vi "E727_StageNavigator.vi"() -> ()   [LabVIEW 2022 SP3]
panel:
  in  "stop":bool
  out "Current position":dbl[](array[numeric]) format="%.6f"
  out "StageRunning":bool
  in  "Repeats":dbl=1.0 min=1.0
  in  "Left x0.5":bool
  in  "Right x0.5":bool
  in  "Up x0.5":bool
  in  "Down x0.5":bool
  in  "Z Resolution (um)":dbl=30.0 min=1.0
  in  "Down Z x4":bool
  in  "Down Z x2":bool
  in  "Up Z x4":bool
  in  "Up Z x2":bool
  in  "Up Z":bool
  in  "Down Z":bool
  in  "Right x4":bool
  in  "Right x2":bool
  in  "Left x4":bool
  in  "Left x2":bool
  in  "Down x4":bool
  in  "Down x2":bool
  in  "Up x4":bool
  in  "Up x2":bool
  in  "StageChannels":string[](array[string])
  in  "On/Off":bool
  in  "X / Y Resolution (um)":dbl=10.0 min=1.0
  in  "Right":bool
  in  "Left":bool
  in  "Up":bool
  in  "Down":bool
  # "STAGE"
  # "Z Focus"
  # "X / Y Navigation"
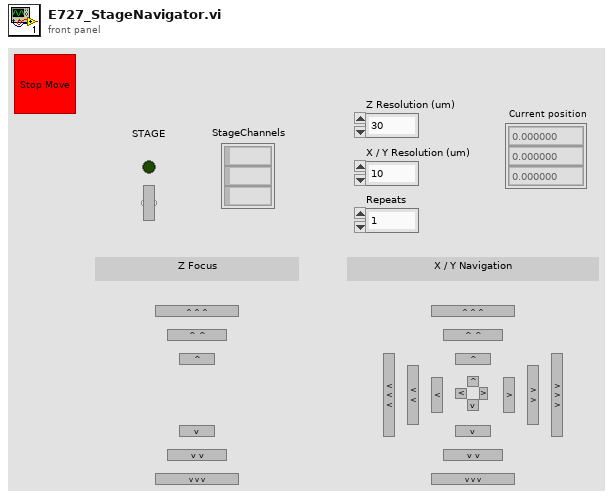
[diagram p1: front panel]
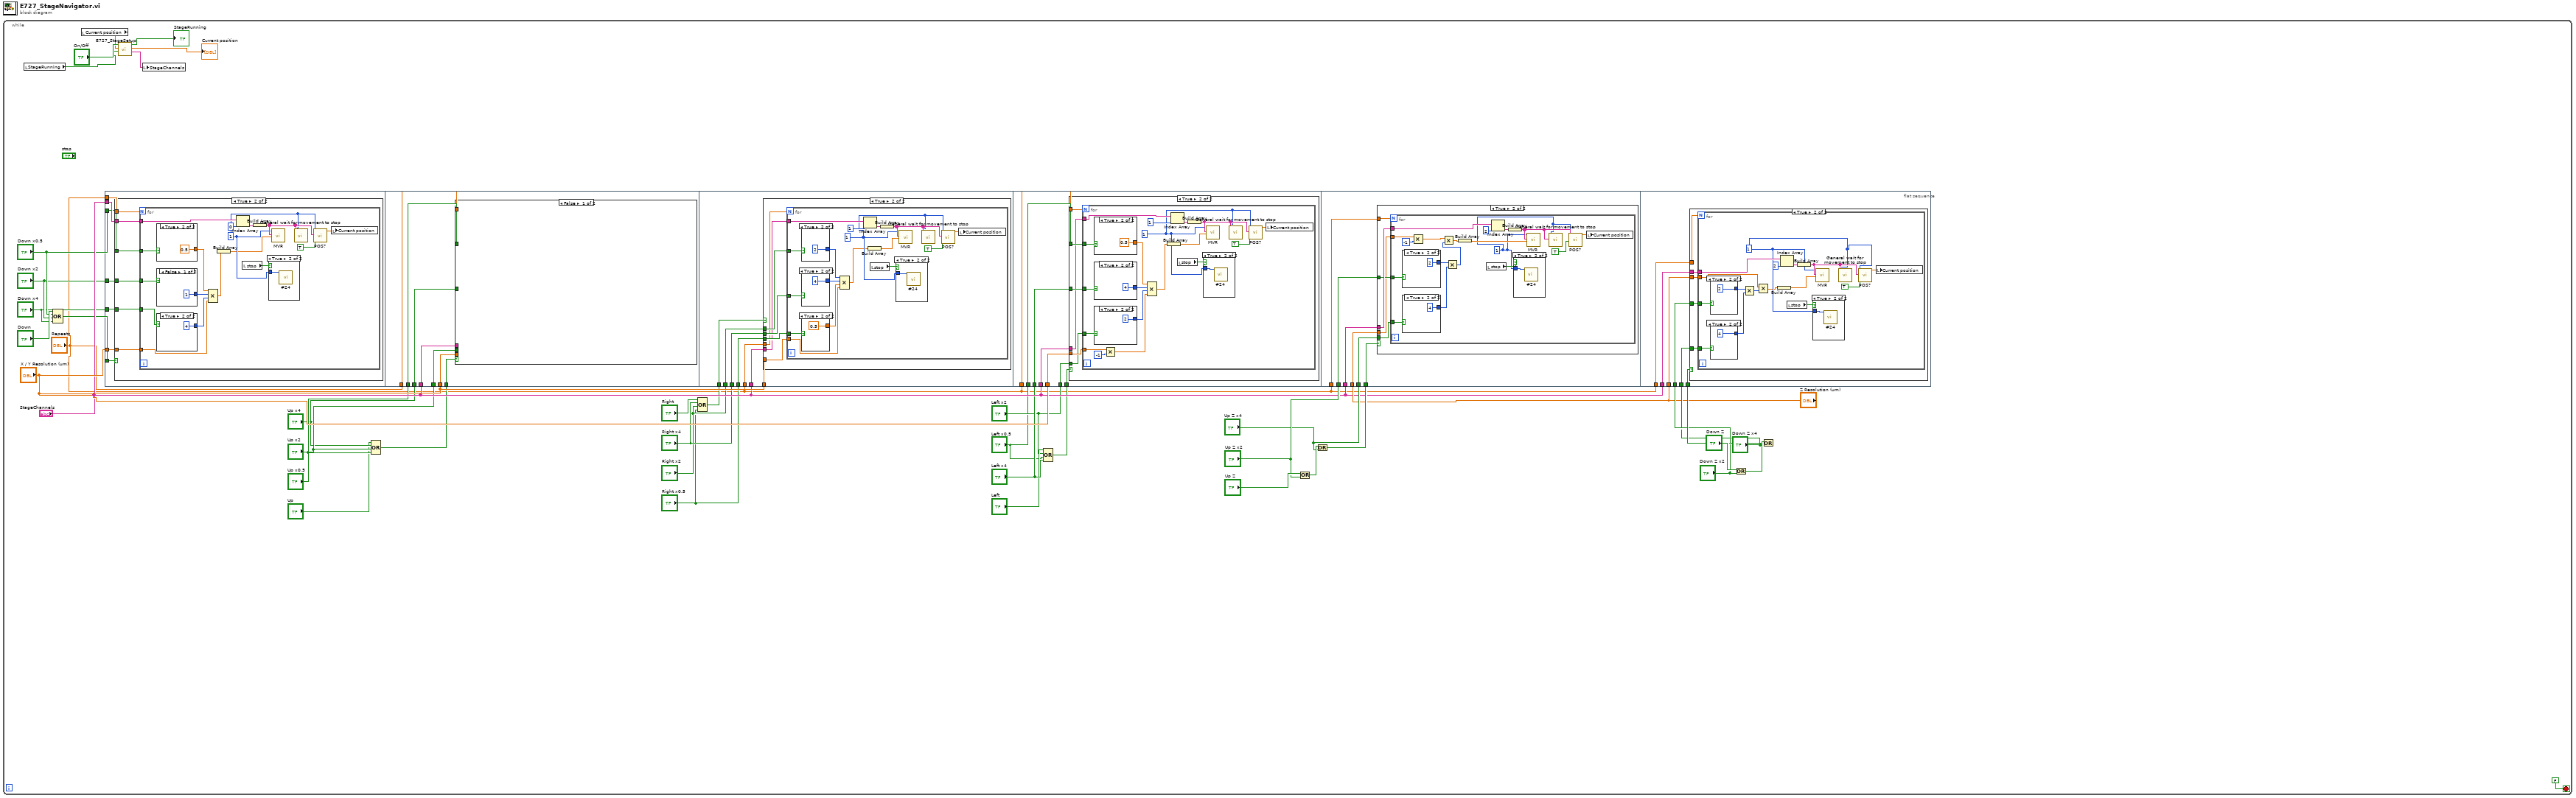
[diagram p0: block diagram]
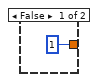
[diagram p4: hidden frame]
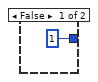
[diagram p5: hidden frame]
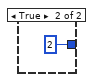
[diagram p6: hidden frame]
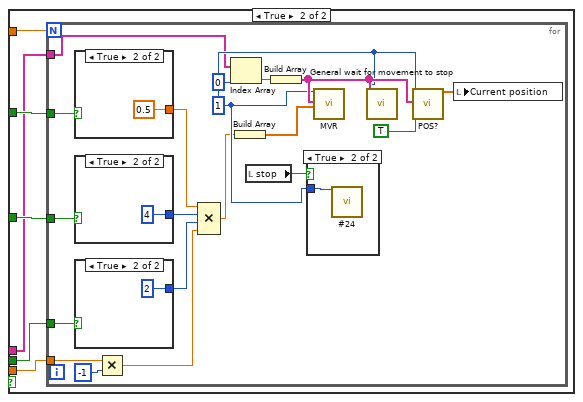
[diagram p7: hidden frame]
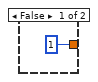
[diagram p9: hidden frame]
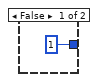
[diagram p10: hidden frame]
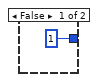
[diagram p11: hidden frame]
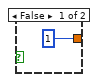
[diagram p14: hidden frame]
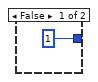
[diagram p15: hidden frame]
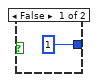
[diagram p16: hidden frame]
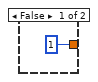
[diagram p19: hidden frame]
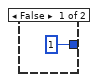
[diagram p20: hidden frame]
diagram:
  n1 = while {
    stop <- FALSE stop-if-true
    n2 = local read "StageRunning"() -> (w5:bool)
    n3 = Compound Arithmetic op=OR("Down", "Down x0.5", "Down x2", "Down x4") -> (w13:bool)
    n4 = local read "Current position"() -> (w1:dbl[])
    n5 = flat-sequence {
      tunnel: "X / Y Resolution (um)" -> [w47]
      tunnel: "StageChannels" -> [w48]
      tunnel: w13 -> [w46]
      tunnel: "Down x2" -> [w45]
      tunnel: "Down x4" -> [w44]
      tunnel: "Down x0.5" -> [w43]
      tunnel: "Repeats" -> [w42]
      tunnel: "X / Y Resolution (um)" -> [w85]
      tunnel: "StageChannels" -> [w84]
      tunnel: "Up x2" -> [w83]
      tunnel: w18 -> [w82]
      tunnel: "Up x4" -> [w81]
      tunnel: "Up x0.5" -> [w80]
      tunnel: "Repeats" -> [w79]
      tunnel: "StageChannels" -> [w124]
      tunnel: "Right x2" -> [w123]
      tunnel: "Right x4" -> [w122]
      tunnel: "X / Y Resolution (um)" -> [w121]
      tunnel: w28 -> [w120]
      tunnel: "Right x0.5" -> [w119]
      tunnel: "Repeats" -> [w118]
      tunnel: "StageChannels" -> [w161]
      tunnel: "X / Y Resolution (um)" -> [w160]
      tunnel: w23 -> [w159]
      tunnel: "Left x4" -> [w158]
      tunnel: "Left x2" -> [w157]
      tunnel: "Left x0.5" -> [w156]
      tunnel: "Repeats" -> [w155]
      tunnel: "StageChannels" -> [w199]
      tunnel: "Z Resolution (um)" -> [w198]
      tunnel: w39 -> [w197]
      tunnel: "Up Z x2" -> [w196]
      tunnel: "Up Z x4" -> [w195]
      tunnel: "Repeats" -> [w194]
      tunnel: "StageChannels" -> [w233]
      tunnel: "Z Resolution (um)" -> [w232]
      tunnel: w33 -> [w231]
      tunnel: "Down Z x2" -> [w230]
      tunnel: "Down Z x4" -> [w229]
      tunnel: "Repeats" -> [w228]
      frame #0 {
        n6 = case shown="True" w46 {
          tunnel: w47 -> [_ w51]
          tunnel: w48 -> [_ w54]
          tunnel: w45 -> [_ w53]
          tunnel: w44 -> [_ w52]
          tunnel: w43 -> [_ w50]
          tunnel: w42 -> [_ w49]
          frame False {
          }
          frame True {
            n7 = for {
              N: w49 -> [_]
              tunnel: w54 -> [w58]
              tunnel: w53 -> [w71]
              tunnel: w52 -> [w70]
              tunnel: w51 -> [w69]
              tunnel: w50 -> [w65]
              w57 = 1 ("System no.")
              n8 = case shown="True" w65 {
                tunnel: [1 0.5] -> w68
                frame False {
                }
                frame True {
                }
              }
              n9 = case shown="False" w71 {
                tunnel: [1 2] -> w66
                frame False {
                }
                frame True {
                }
              }
              n10 = case shown="True" w70 {
                tunnel: [1 4] -> w67
                frame False {
                }
                frame True {
                }
              }
              n11 = Compound Arithmetic op=MULTIPLY(w68, w66, w67, w69) -> (w56:dbl)
              n12 = Build Array(w56) -> (w55:dbl[])
              n13 = Index Array(array=w58, index=0) -> (element=w61:string)
              n14 = local read "stop"() -> (w62:bool)
              n15 = Build Array(w61) -> (w63:string[])
              n16 = case shown="True" w62 {
                tunnel: w57 -> [_ w72]
                frame False {
                }
                frame True {
                  n17 = call "#24.vi"("System no."=w72) -> ()  [unwired: 1 in, 18 out]
                }
              }
              n18 = call "MVR.vi"("System no."=w57, "Axes to move"=w63, "Position values"=w55) -> ()  [unwired: 2 in, 15 out]
              n19 = call "General wait for movement to stop.vi"("System no."=w57, "Axes to wait for"=w63) -> ()  [unwired: 6 in, 12 out]
              n20 = call "POS?.vi"("System no."=w57, "Axes to query"=w63, "All axes?"=TRUE) -> ("Position"=w64:dbl[])  [unwired: 2 in, 14 out]
              n21 = local write "Current position"(w64) -> ()
            }
          }
        }
      }
      frame #1 {
        n22 = case shown="False" w82 {
          tunnel: w85 -> [_ w91]
          tunnel: w84 -> [_ w87]
          tunnel: w83 -> [_ w90]
          tunnel: w81 -> [_ w89]
          tunnel: w80 -> [_ w88]
          tunnel: w79 -> [_ w86]
          frame False {
          }
          frame True {
            n23 = for {
              N: w86 -> [_]
              tunnel: w91 -> [w102]
              tunnel: w90 -> [w109]
              tunnel: w89 -> [w108]
              tunnel: w88 -> [w103]
              tunnel: w87 -> [w94]
              w95 = 1 ("System no.")
              n24 = case shown="True" w103 {
                tunnel: [1 0.5] -> w106
                frame False {
                }
                frame True {
                }
              }
              n25 = case shown="True" w108 {
                tunnel: [1 4] -> w105
                frame False {
                }
                frame True {
                }
              }
              n26 = case shown="True" w109 {
                tunnel: [1 2] -> w104
                frame False {
                }
                frame True {
                }
              }
              n27 = Multiply(x=w102, y=-1) -> (x*y=w107:dbl)
              n28 = Compound Arithmetic op=MULTIPLY(w106, w105, w104, w107) -> (w92:dbl)
              n29 = Index Array(array=w94, index=0) -> (element=w98:string)
              n30 = Build Array(w92) -> (w93:dbl[])
              n31 = local read "stop"() -> (w99:bool)
              n32 = Build Array(w98) -> (w100:string[])
              n33 = case shown="True" w99 {
                tunnel: w95 -> [_ w111]
                frame False {
                }
                frame True {
                  n34 = call "#24.vi"("System no."=w111) -> ()  [unwired: 1 in, 18 out]
                }
              }
              n35 = call "MVR.vi"("System no."=w95, "Axes to move"=w100, "Position values"=w93) -> ()  [unwired: 2 in, 15 out]
              n36 = call "General wait for movement to stop.vi"("System no."=w95, "Axes to wait for"=w100) -> ()  [unwired: 6 in, 12 out]
              n37 = call "POS?.vi"("System no."=w95, "Axes to query"=w100, "All axes?"=TRUE) -> ("Position"=w101:dbl[])  [unwired: 2 in, 14 out]
              n38 = local write "Current position"(w101) -> ()
            }
          }
        }
      }
      frame #2 {
        n39 = case shown="True" w120 {
          tunnel: w121 -> [_ w127]
          tunnel: w124 -> [_ w126]
          tunnel: w123 -> [_ w130]
          tunnel: w122 -> [_ w129]
          tunnel: w119 -> [_ w128]
          tunnel: w118 -> [_ w125]
          frame False {
          }
          frame True {
            n40 = for {
              N: w125 -> [_]
              tunnel: w130 -> [w147]
              tunnel: w129 -> [w146]
              tunnel: w128 -> [w144]
              tunnel: w127 -> [w141]
              tunnel: w126 -> [w135]
              w133 = 1 ("System no.")
              n41 = case shown="True" w147 {
                tunnel: [1 2] -> w143
                frame False {
                }
                frame True {
                }
              }
              n42 = case shown="True" w146 {
                tunnel: [1 4] -> w142
                frame False {
                }
                frame True {
                }
              }
              n43 = case shown="True" w144 {
                tunnel: [1 0.5] -> w145
                frame False {
                }
                frame True {
                }
              }
              n44 = Compound Arithmetic op=MULTIPLY(w143, w142, w145, w141) -> (w131:dbl)
              n45 = Index Array(array=w135, index=1) -> (element=w137:string)
              n46 = Build Array(w131) -> (w132:dbl[])
              n47 = local read "stop"() -> (w138:bool)
              n48 = Build Array(w137) -> (w139:string[])
              n49 = case shown="True" w138 {
                tunnel: w133 -> [_ w148]
                frame False {
                }
                frame True {
                  n50 = call "#24.vi"("System no."=w148) -> ()  [unwired: 1 in, 18 out]
                }
              }
              n51 = call "MVR.vi"("System no."=w133, "Axes to move"=w139, "Position values"=w132) -> ()  [unwired: 2 in, 15 out]
              n52 = call "General wait for movement to stop.vi"("System no."=w133, "Axes to wait for"=w139) -> ()  [unwired: 6 in, 12 out]
              n53 = call "POS?.vi"("System no."=w133, "Axes to query"=w139, "All axes?"=TRUE) -> ("Position"=w140:dbl[])  [unwired: 2 in, 14 out]
              n54 = local write "Current position"(w140) -> ()
            }
          }
        }
      }
      frame #3 {
        n55 = case shown="True" w159 {
          tunnel: w160 -> [_ w167]
          tunnel: w161 -> [_ w163]
          tunnel: w157 -> [_ w166]
          tunnel: w158 -> [_ w165]
          tunnel: w156 -> [_ w164]
          tunnel: w155 -> [_ w162]
          frame False {
          }
          frame True {
            n56 = for {
              N: w162 -> [_]
              tunnel: w167 -> [w186]
              tunnel: w166 -> [w184]
              tunnel: w165 -> [w183]
              tunnel: w164 -> [w178]
              tunnel: w163 -> [w171]
              w170 = 1 ("System no.")
              n57 = case shown="True" w178 {
                tunnel: [1 0.5] -> w182
                frame False {
                }
                frame True {
                }
              }
              n58 = case shown="True" w183 {
                tunnel: [1 4] -> w180
                frame False {
                }
                frame True {
                }
              }
              n59 = case shown="True" w184 {
                tunnel: [1 2] -> w179
                frame False {
                }
                frame True {
                }
              }
              n60 = Multiply(x=w186, y=-1) -> (x*y=w181:dbl)
              n61 = Compound Arithmetic op=MULTIPLY(w182, w180, w179, w181) -> (w168:dbl)
              n62 = Build Array(w168) -> (w169:dbl[])
              n63 = Index Array(array=w171, index=1) -> (element=w174:string)
              n64 = local read "stop"() -> (w175:bool)
              n65 = Build Array(w174) -> (w176:string[])
              n66 = case shown="True" w175 {
                tunnel: w170 -> [_ w187]
                frame False {
                }
                frame True {
                  n67 = call "#24.vi"("System no."=w187) -> ()  [unwired: 1 in, 18 out]
                }
              }
              n68 = call "MVR.vi"("System no."=w170, "Axes to move"=w176, "Position values"=w169) -> ()  [unwired: 2 in, 15 out]
              n69 = call "General wait for movement to stop.vi"("System no."=w170, "Axes to wait for"=w176) -> ()  [unwired: 6 in, 12 out]
              n70 = call "POS?.vi"("System no."=w170, "Axes to query"=w176, "All axes?"=TRUE) -> ("Position"=w177:dbl[])  [unwired: 2 in, 14 out]
              n71 = local write "Current position"(w177) -> ()
            }
          }
        }
      }
      frame #4 {
        n72 = case shown="True" w197 {
          tunnel: w198 -> [_ w201]
          tunnel: w199 -> [_ w204]
          tunnel: w196 -> [_ w203]
          tunnel: w195 -> [_ w202]
          tunnel: w194 -> [_ w200]
          frame False {
          }
          frame True {
            n73 = for {
              N: w200 -> [_]
              tunnel: w204 -> [w208]
              tunnel: w203 -> [w219]
              tunnel: w202 -> [w218]
              tunnel: w201 -> [w215]
              w205 = 1 ("System no.")
              n74 = case shown="True" w219 {
                tunnel: [1 2] -> w221
                frame False {
                }
                frame True {
                }
              }
              n75 = case shown="True" w218 {
                tunnel: [1 4] -> w222
                frame False {
                }
                frame True {
                }
              }
              n76 = Multiply(x=w215, y=-1) -> (x*y=w216:dbl)
              n77 = Multiply(x=w221, y=w222) -> (x*y=w220:i32)
              n78 = Multiply(x=w216, y=w220) -> (x*y=w207:dbl)
              n79 = Build Array(w207) -> (w206:dbl[])
              n80 = local read "stop"() -> (w212:bool)
              n81 = Index Array(array=w208, index=2) -> (element=w211:string)
              n82 = Build Array(w211) -> (w213:string[])
              n83 = case shown="True" w212 {
                tunnel: w205 -> [_ w223]
                frame False {
                }
                frame True {
                  n84 = call "#24.vi"("System no."=w223) -> ()  [unwired: 1 in, 18 out]
                }
              }
              n85 = call "MVR.vi"("System no."=w205, "Axes to move"=w213, "Position values"=w206) -> ()  [unwired: 2 in, 15 out]
              n86 = call "General wait for movement to stop.vi"("System no."=w205, "Axes to wait for"=w213) -> ()  [unwired: 6 in, 12 out]
              n87 = call "POS?.vi"("System no."=w205, "Axes to query"=w213, "All axes?"=TRUE) -> ("Position"=w214:dbl[])  [unwired: 2 in, 14 out]
              n88 = local write "Current position"(w214) -> ()
            }
          }
        }
      }
      frame #5 {
        n89 = case shown="True" w231 {
          tunnel: w232 -> [_ w237]
          tunnel: w233 -> [_ w238]
          tunnel: w230 -> [_ w236]
          tunnel: w229 -> [_ w235]
          tunnel: w228 -> [_ w234]
          frame False {
          }
          frame True {
            n90 = for {
              N: w234 -> [_]
              tunnel: w238 -> [w242]
              tunnel: w237 -> [w251]
              tunnel: w236 -> [w250]
              tunnel: w235 -> [w249]
              w241 = 1 ("System no.")
              n91 = case shown="True" w250 {
                tunnel: [1 2] -> w253
                frame False {
                }
                frame True {
                }
              }
              n92 = case shown="True" w249 {
                tunnel: [1 4] -> w254
                frame False {
                }
                frame True {
                }
              }
              n93 = Multiply(x=w253, y=w254) -> (x*y=w252:i32)
              n94 = Multiply(x=w251, y=w252) -> (x*y=w240:dbl)
              n95 = Build Array(w240) -> (w239:dbl[])
              n96 = Index Array(array=w242, index=2) -> (element=w245:string)
              n97 = local read "stop"() -> (w246:bool)
              n98 = Build Array(w245) -> (w247:string[])
              n99 = case shown="True" w246 {
                tunnel: w241 -> [_ w255]
                frame False {
                }
                frame True {
                  n100 = call "#24.vi"("System no."=w255) -> ()  [unwired: 1 in, 18 out]
                }
              }
              n101 = call "MVR.vi"("System no."=w241, "Axes to move"=w247, "Position values"=w239) -> ()  [unwired: 2 in, 15 out]
              n102 = call "General wait for movement to stop.vi"("System no."=w241, "Axes to wait for"=w247) -> ()  [unwired: 6 in, 12 out]
              n103 = call "POS?.vi"("System no."=w241, "Axes to query"=w247, "All axes?"=TRUE) -> ("Position"=w248:dbl[])  [unwired: 2 in, 14 out]
              n104 = local write "Current position"(w248) -> ()
            }
          }
        }
      }
    }
    n105 = call "E727_StageSetup.vi"("StageRunningIn"=w5, "Position 2"=w1, "StageOn/Off"="On/Off") -> ("StageChannels"=w4:string[], "Current position"=→"Current position":dbl[], "StageRunningOut"=→"StageRunning":bool)  [unwired: 5 in, 1 out]
    n106 = local write "StageChannels"(w4) -> ()
    n107 = Compound Arithmetic op=OR("Up", "Up x4", "Up x2", "Up x0.5") -> (w18:bool)
    n108 = Compound Arithmetic op=OR("Right", "Right x4", "Right x2", "Right x0.5") -> (w28:bool)
    n109 = Compound Arithmetic op=OR("Left", "Left x2", "Left x0.5", "Left x4") -> (w23:bool)
    n110 = Or(x="Up Z", y="Up Z x2") -> (x .or. y?=w41:bool)
    n111 = Or(x=w41, y="Up Z x4") -> (x .or. y?=w39:bool)
    n112 = Or(x="Down Z", y="Down Z x2") -> (x .or. y?=w35:bool)
    n113 = Or(x=w35, y="Down Z x4") -> (x .or. y?=w33:bool)
  }
